vi "LOER_GetTerms.vi"(0 "XRef":T12, 1 "State In":T10={"Inputs"=1, "SelectedIndex"=1, "ClassInfo"=[], "Width"=100, "EventReg Type"=variant}) -> (14 "Terms":T2, 15 "Fatal Error Out":T1)   [LabVIEW 2016, in "LV Object Event Registration Node.xnode"]
uses:
  LV Object Event Registration Node.xnode
  <vilib>/XNodeSupport/XNodeXNodeRef.ctl
  LOER_State.ctl
  LOER_ClassInfo.ctl
  <vilib>/XNodeSupport/XNodeTerm4Array.ctl
  <vilib>/XNodeSupport/XNodeTerm4.ctl
  <vilib>/XNodeSupport/XNodeString.ctl
  <vilib>/XNodeSupport/XNodeVariant.ctl
  <vilib>/XNodeSupport/XNodeRect32.ctl
  <vilib>/XNodeSupport/XNodeInt.ctl
  <vilib>/XNodeSupport/XNodeBool.ctl
  <vilib>/XNodeSupport/XNodeTermDirection.ctl
  <vilib>/XNodeSupport/XNodeErrorCluster.ctl
  <vilib>/XNodeSupport/NI_XNodeSupport.lvlib
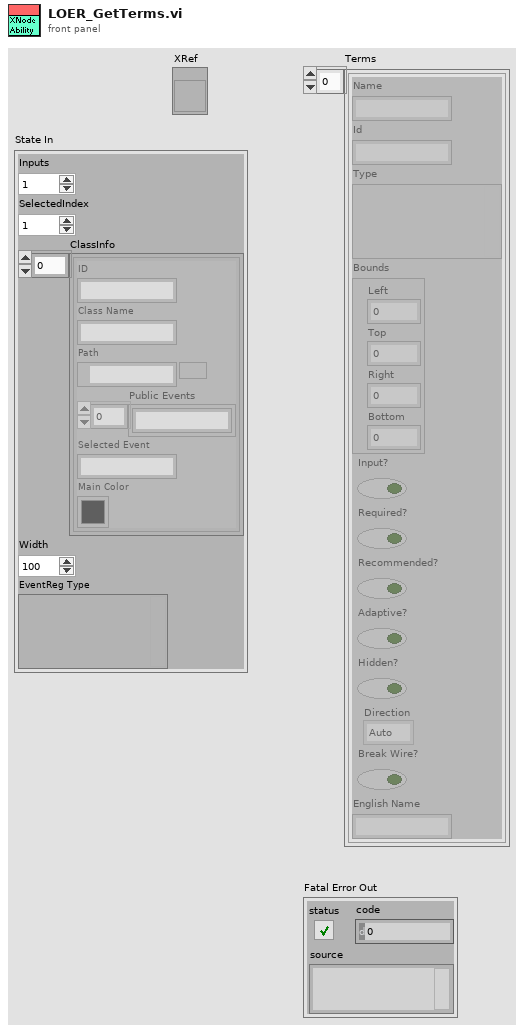
[diagram p1: front panel]
types:
  T1 = typedef "NI_XNodeSupport.lvlib/XNodeErrorCluster.ctl" = errorcluster
  T2 = typedef "NI_XNodeSupport.lvlib/XNodeTerm4Array.ctl" = T3[]
  T3 = typedef "NI_XNodeSupport.lvlib/XNodeTerm4.ctl" = cluster{"Name":T4, "Id":T4, "Type":T5, "Bounds":T6, "Input?":T8, "Required?":T8, "Recommended?":T8, "Adaptive?":T8, "Hidden?":T8, "Direction":T9, "Break Wire?":T8, "English Name":T4}
  T4 = typedef "NI_XNodeSupport.lvlib/XNodeString.ctl" = string
  T5 = typedef "NI_XNodeSupport.lvlib/XNodeVariant.ctl" = variant
  T6 = typedef "NI_XNodeSupport.lvlib/XNodeRect32.ctl" = cluster{"Left":T7, "Top":T7, "Right":T7, "Bottom":T7}
  T7 = typedef "NI_XNodeSupport.lvlib/XNodeInt.ctl" = i32
  T8 = typedef "NI_XNodeSupport.lvlib/XNodeBool.ctl" = bool
  T9 = typedef "NI_XNodeSupport.lvlib/XNodeTermDirection.ctl" = enum32{"Auto", "Up", "Down", "Left", "Right", "Center"}
  T10 = typedef "LV Object Event Registration Node.xnode/LOER_State.ctl" = cluster{"Inputs":u16, "SelectedIndex":i16, "ClassInfo":T11[], "Width":u16, "EventReg Type":variant}
  T11 = typedef "LV Object Event Registration Node.xnode/LOER_ClassInfo.ctl" = cluster{"ID":string, "Class Name":string, "Path":path, "Public Events":string[], "Selected Event":string, "Main Color":u32}
  T12 = typedef "NI_XNodeSupport.lvlib/XNodeXNodeRef.ctl" = refnum<vi>
  T13 = typedef "NI_XNodeSupport.lvlib/XNodeBounds.ctl" = cluster{"Width":T7, "Height":T7}
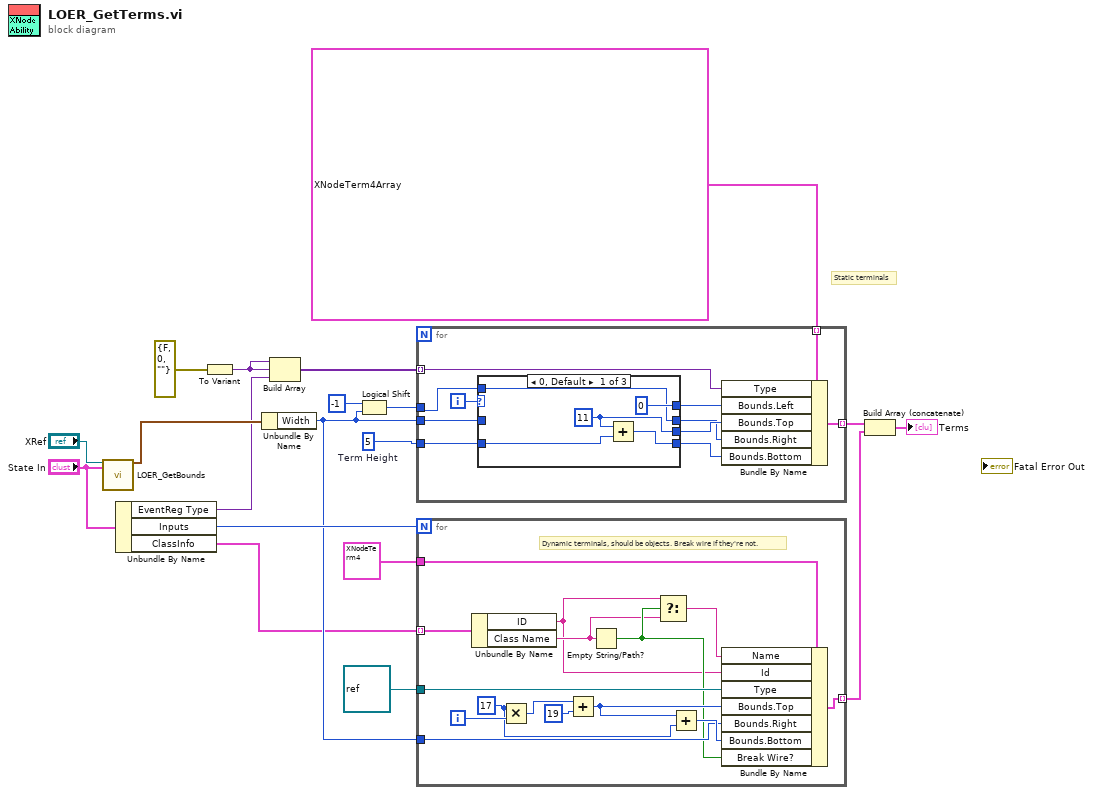
[diagram p0: block diagram]
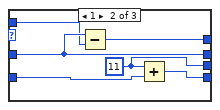
[diagram p2: hidden frame]
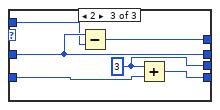
[diagram p3: hidden frame]
diagram:
  w6 = 5  # Term Height
  # "Static terminals"
  n1 = call "LOER_GetBounds.vi"("XRef"="XRef", "State In"="State In") -> ("Bounds"=w14:T13)  [unwired: 16 in, 1 out]
  n2 = Unbundle By Name("State In") -> ("EventReg Type"=w1:variant, "Inputs"=w12:u16, "ClassInfo"=w2:T11[])
  n3 = To Variant(anything=errorcluster {"status"=FALSE, "code"=0, "source"=""} ("error in (no error)")) -> (Variant=w17:variant)
  n4 = Unbundle By Name(w14) -> ("Width"=w5:T7)
  n5 = Build Array(w17, w17, w1) -> (w16:variant[])
  n6 = Logical Shift(y=i16 -1, x=w5) -> (x << y=w3:T7)
  n7 = for {
    tunnel: T2 [{"Name"="Error In", "Id"="error in", "Type"=variant, "Bounds"={"Left"=0, "Top"=0, "Right"=0, "Bottom"=0}, "Input?"=TRUE, "Required?"=FALSE, "Recommended?"=FALSE, "Adaptive?"=FALSE, "Hidden?"=FALSE, "Direction"=enum."Auto", "Break Wire?"=FALSE, "English Name"=""}, {"Name"="Error Out", "Id"="error out", "Type"=variant, "Bounds"={"Left"=0, "Top"=0, "Right"=0, "Bottom"=0}, "Input?"=FALSE, "Required?"=FALSE, "Recommended?"=TRUE, "Adaptive?"=FALSE, "Hidden?"=FALSE, "Direction"=enum."Auto", "Break Wire?"=FALSE, "English Name"=""}, {"Name"="Event Registration Refnum", "Id"="Object Event Reg", "Type"=variant, "Bounds"={"Left"=0, "Top"=0, "Right"=0, "Bottom"=0}, "Input?"=FALSE, "Required?"=FALSE, "Recommended?"=TRUE, "Adaptive?"=TRUE, "Hidden?"=FALSE, "Direction"=enum."Auto", "Break Wire?"=FALSE, "English Name"=""}] ("Terms") -> [w30] mode=indexing
    tunnel: w16 -> [w29] mode=indexing
    tunnel: [w28] -> w9 mode=indexing
    tunnel: w5 -> [w22]
    tunnel: w6 -> [w21]
    tunnel: w3 -> [w20]
    i -> [w27]
    n8 = case shown="0, Default" w27 {
      tunnel: [T7 0 ("Bounds.Left") w40 w46] -> w26
      tunnel: [w34 w39 w45] -> w25
      tunnel: [w31 w41 w47] -> w24
      tunnel: [w32 w37 w43] -> w23
      tunnel: w22 -> [_ w41 w47]
      tunnel: w21 -> [w33 w38 w44]
      tunnel: w20 -> [w31 w36 w42]
      frame 0, Default {
        w34 = T7 11 ("Bounds.Left")
        n9 = Add(x=w34, y=w33) -> (x+y=w32:T7)
      }
      frame 1 {
        w39 = T7 11 ("Bounds.Left")
        n10 = Subtract(x=w41, y=w36) -> (x-y=w40:T7)
        n11 = Add(x=w39, y=w38) -> (x+y=w37:T7)
      }
      frame 2 {
        w45 = T7 3 ("Bounds.Left")
        n12 = Subtract(x=w47, y=w42) -> (x-y=w46:T7)
        n13 = Add(x=w45, y=w44) -> (x+y=w43:T7)
      }
    }
    n14 = Bundle By Name(cluster=w30, "Type"=w29, "Bounds.Left"=w26, "Bounds.Top"=w25, "Bounds.Right"=w24, "Bounds.Bottom"=w23) -> (w28:T3)
  }
  n15 = for {
    N: w12 -> [_]
    tunnel: T3 {"Name"="Event", "Id"="Event", "Type"=variant, "Bounds"={"Left"=0, "Top"=0, "Right"=4, "Bottom"=0}, "Input?"=TRUE, "Required?"=TRUE, "Recommended?"=FALSE, "Adaptive?"=TRUE, "Hidden?"=FALSE, "Direction"=enum."Auto", "Break Wire?"=FALSE, "English Name"=""} ("Term 4") -> [w62]
    tunnel: refnum<class> refnum ("LabVIEW Object") -> [w61]
    tunnel: [w60] -> w8 mode=indexing
    tunnel: w5 -> [w55]
    tunnel: w2 -> [w54] mode=indexing
    i -> [w58]
    w52 = 17
    # "Dynamic terminals, should be objects. Break wire if they're not."
    n16 = Unbundle By Name(w54) -> ("ID"=w48:string, "Class Name"=w50:string)
    n17 = Multiply(x=w52, y=w58) -> (x*y=w57:i32)
    n18 = Add(x=w57, y=19) -> (x+y=w53:i32)
    n19 = Empty String/Path?(string/path=w50) -> (empty?=w51:bool)
    n20 = Select(t=w48, s=w51, f=w50) -> (s? t:f=w49:string)
    n21 = Add(x=w53, y=w52) -> (x+y=w56:i32)
    n22 = Bundle By Name(cluster=w62, "Name"=w49, "Id"=w48, "Type"=w61, "Bounds.Top"=w53, "Bounds.Right"=w55, "Bounds.Bottom"=w56, "Break Wire?"=w51) -> (w60:T3)
  }
  n23 = Build Array (concatenate)(w9, w8) -> (→"Terms":T3[])
